vi "SGLtoI16 Array.vi"(9 "Input Valid":bool, 10 "Input":sgl[](array[numeric])=[0.0, 0.0, 0.0, 0.0]) -> (1 "Output Valid":bool, 2 "Output":i16[](array[numeric]))   [LabVIEW 2014]
panel:
  # "Copyright 2014 Vidrio Technologies\nScanImage 5 software is licensed under the Apache License, Version 2.0 (the \"License\"); you may not use any files contained\nwithin the ScanImage 5 release except in compliance with the License. You may obtain a copy of the License at\n http://www.apache.org/licenses/LICENSE-2.0\nUnless required by applicable law or agreed to in writing, software distributed under the License is distributed on an\n\"AS IS\" BASIS, WITHOUT WARRANTIES OR CONDITIONS OF ANY KIND, either express or implied. See the License for the\n specific language governing permissions and limitations under the License."
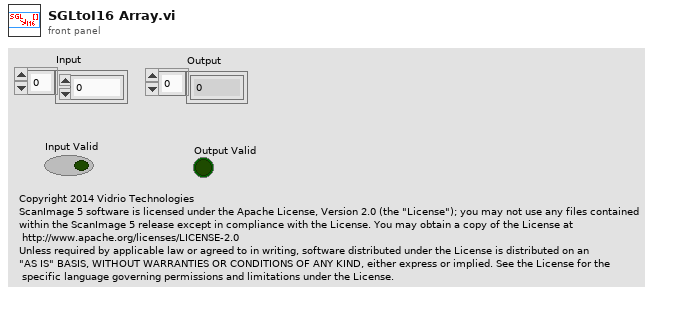
[diagram p1: front panel]
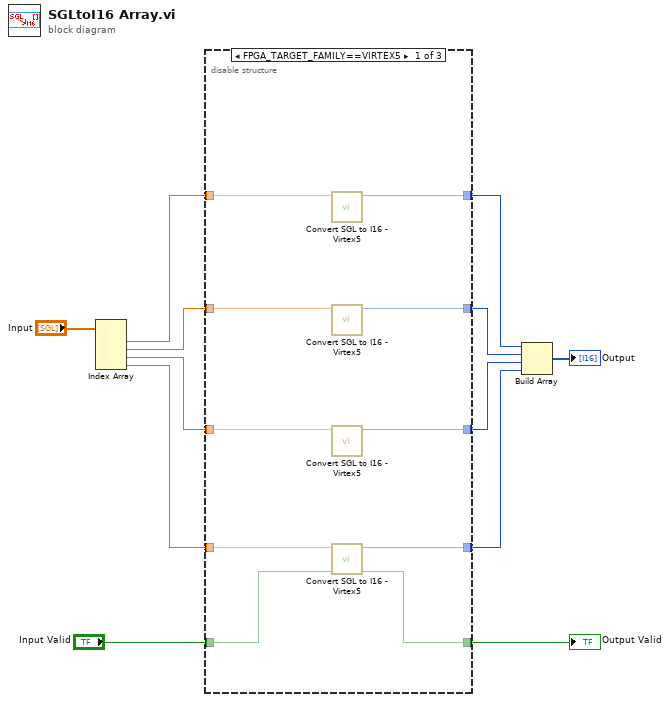
[diagram p0: block diagram]
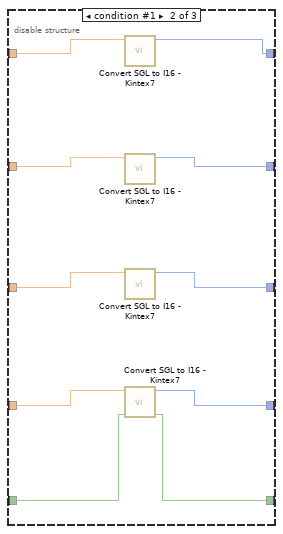
[diagram p2: hidden frame]
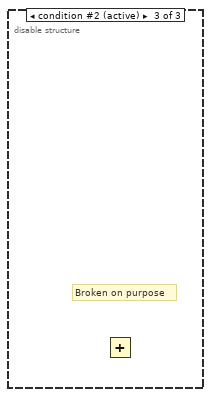
[diagram p3: hidden frame]
diagram:
  n1 = Index Array(array="Input") -> (element #1=w9:sgl, element #2=w8:sgl, element #3=w7:sgl, element #4=w6:sgl)  [unwired: 4 in]
  n2 = disable-structure shown="FPGA_TARGET_FAMILY==VIRTEX5" {
    disable-tunnel: "Input Valid" -> [w14 w24 _]
    disable-tunnel: [w13 w23 _] -> w11
    disable-tunnel: w9 -> [w22 w32 _]
    disable-tunnel: w8 -> [w20 w30 _]
    disable-tunnel: w7 -> [w18 w28 _]
    disable-tunnel: w6 -> [w16 w26 _]
    disable-tunnel: [w21 w31 _] -> w5
    disable-tunnel: [w19 w29 _] -> w4
    disable-tunnel: [w17 w27 _] -> w3
    disable-tunnel: [w15 w25 _] -> w2
    frame condition #0 {
      n3 = call "Convert SGL to I16 - Virtex5.vi"("Data In"=w22) -> ("Data Out"=w21:i16)  [unwired: 8 in, 1 out]
      n4 = call "Convert SGL to I16 - Virtex5.vi"("Data In"=w20) -> ("Data Out"=w19:i16)  [unwired: 8 in, 1 out]
      n5 = call "Convert SGL to I16 - Virtex5.vi"("Data In"=w18) -> ("Data Out"=w17:i16)  [unwired: 8 in, 1 out]
      n6 = call "Convert SGL to I16 - Virtex5.vi"("Data In"=w16, "Data Valid In"=w14) -> ("Data Out"=w15:i16, "Data Valid Out"=w13:bool)  [unwired: 7 in]
    }
    frame condition #1 {
      n7 = call "Convert SGL to I16 - Kintex7.vi"("Data In"=w32) -> ("Data Out"=w31:i16)  [unwired: 8 in, 1 out]
      n8 = call "Convert SGL to I16 - Kintex7.vi"("Data In"=w30) -> ("Data Out"=w29:i16)  [unwired: 8 in, 1 out]
      n9 = call "Convert SGL to I16 - Kintex7.vi"("Data In"=w28) -> ("Data Out"=w27:i16)  [unwired: 8 in, 1 out]
      n10 = call "Convert SGL to I16 - Kintex7.vi"("Data In"=w26, "Data Valid In"=w24) -> ("Data Out"=w25:i16, "Data Valid Out"=w23:bool)  [unwired: 7 in]
    }
    frame condition #2 (active) {
      # "Broken on purpose"
      n11 = Add() -> ()  [unwired: 2 in, 1 out]
    }
  }
  "Output Valid" <- w11
  n12 = Build Array(w5, w4, w3, w2) -> (→"Output":i16[])
